vi "global value 15 b.vi"() -> ()   [LabVIEW 2025]
uses:
  Global 2.vi
panel:
  out "c":dbl
  out "b":dbl
  out "a":dbl
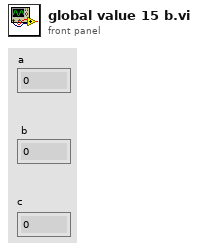
[diagram p1: front panel]
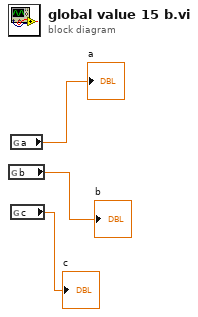
[diagram p0: block diagram]
diagram:
  n1 = global read "Global 2.vi" "b"() -> (→"b":dbl)
  n2 = global read "Global 2.vi" "a"() -> (→"a":dbl)
  n3 = global read "Global 2.vi" "c"() -> (→"c":dbl)
